vi "6.Move.vi"() -> ()   [LabVIEW 2017]
uses:
  <vilib>/robotics/Steering/Wheel/Wheel Parameters.ctl
  <vilib>/robotics/Steering/Wheel/Rotation Direction.ctl
  <vilib>/robotics/Steering/Differential Steering Frame/NI_Robotics_Differential Steering Frame.lvclass
  E:/National Instruments/LabVIEW 2017/vi.lib/robotics/Steering/Steering Frame/NI_Robotics_Steering Frame.lvclass
  <vilib>/robotics/Steering/Fixed Wheel/Create Fixed Wheel.vi
  <vilib>/robotics/Steering/Differential Steering Frame/Create Differential Steering Frame.vi
  <vilib>/robotics/Steering/Steering Frame/Apply Steering Frame Velocity to Motors.vi
  <vilib>/robotics/Steering/Create Steering Frame/NI_Robotics_Create Steering Frame.xnode
  <vilib>/robotics/Steering/Class Type Definitions/Differential Steering Frame.ctl
  <vilib>/robotics/Steering/Class Type Definitions/NI_Robotics_Steering Class Types.lvlib
  <vilib>/robotics/Steering/Fixed Wheel/NI_Robotics_Fixed Wheel.lvclass
  <vilib>/robotics/Steering/Wheel/NI_Robotics_Wheel.lvclass
  <vilib>/robotics/Steering/Steering Frame/NI_Robotics_Steering Frame.lvclass
  E:/National Instruments/LabVIEW 2017/vi.lib/robotics/Steering/Special Steering Frame/NI_Robotics_Special Steering Frame.lvclass
panel:
  in  "停止":bool
  out "每个轮子的矢量速度":dbl[](array[numeric])
  in  "坐标系下的X、Y、θ的速度":dbl[](array[numeric])=[0.0, 0.0, 0.0]
  # "X（cm）\nY（cm）\nθ（弧度）"
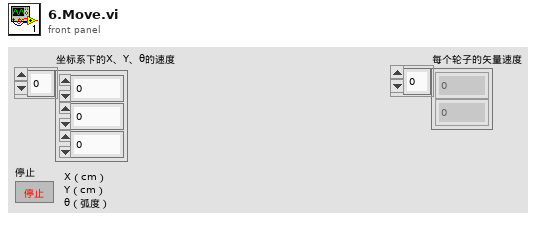
[diagram p1: front panel]
types:
  T1 = typedef "NI_Robotics_Steering Class Types.lvlib/Differential Steering Frame.ctl" = refnum<class "NI_Robotics_Differential Steering Frame.lvclass">
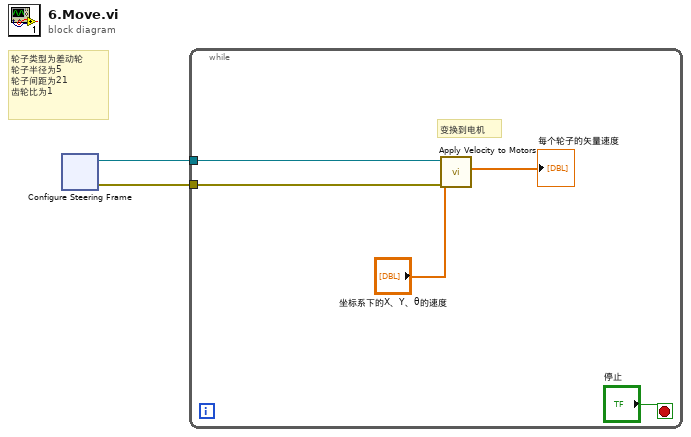
[diagram p0: block diagram]
diagram:
  # "轮子类型为差动轮\n轮子半径为5\n轮子间距为21\n齿轮比为1"
  n1 = xnode ("Configure Steering Frame")() -> ("differential steering frame out"=w1:T1, "error out"=w2:errorcluster)  [unwired: 1 in]
  n2 = while {
    tunnel: w2 -> [w5]
    tunnel: w1 -> [w4]
    stop <- "停止" stop-if-true
    # "变换到电机"
    n3 = call-poly <vilib>:"Apply Velocity to Motors.vi"("error in (no error)"=w5, "steering frame velocity"="坐标系下的X、Y、θ的速度", "steering frame in"=w4) -> ("ccw motor velocity setpoints"=→"每个轮子的矢量速度":dbl[])  [unwired: 4 in, 4 out]
  }
